vi "MCSQH.vi"(8 "TimeStamp":u32, 10 "activePMT":u8) -> (0 "MCSWriteTimeout":bool)   [LabVIEW 2014]
uses:
  <vilib>/rvi/Emulation/niFpgaSctlEmulationGetInTimedLoop.vi
  <vilib>/rvi/interface/RandomDataEmulation/niFpgaRandomDataHandleErrors.vi
  queueHandlerGlobals.vi
  <vilib>/rvi/Emulation/niFpgaProcessEmulError.vi
  <vilib>/rvi/DataTransferAndStorage/Container/XNode/niFpgaContainer.xnode
  <vilib>/rvi/interface/RandomDataEmulation/nirviRandomDataFpgaReadWriteTemplate.vi
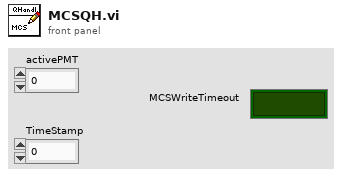
[diagram p1: front panel]
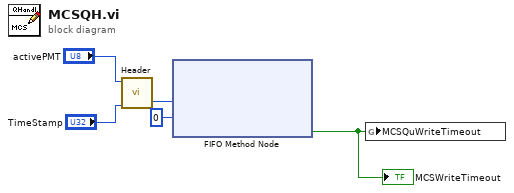
[diagram p0: block diagram]
diagram:
  n1 = call "Header.vi"("23BitData"="TimeStamp", "8BitHead"="activePMT") -> ("32BitOutput"=w5:u32)  [unwired: 3 in]
  n2 = xnode ("FIFO Method Node")("Element"=w5, "Timeout"=0) -> ("Timed Out?"=w1:bool)  [unwired: 1 in, 1 out]
  "MCSWriteTimeout" <- w1
  n3 = global write "queueHandlerGlobals.vi" "MCSQuWriteTimeout"(w1) -> ()
